vi "AbortMultiple.vi"(8 "error in (no error)":errorcluster, 9 "taskId":i32(ring) items=["TLibrary", "T01", "T02", "T03", "T04", "T05", "T06", "T07", "T08", "T09", "T10", "T11", "T12", "T13", "T14", "T15", "T16", "T17", "T18", "T19", "T20", "T21", "T22", "T23", "T24", "T25", "T26", "T27", "T28", "T29", "T30", "T31"], 10 "axis names":string[](array[string]), 11 "controller in":refnum<k24>) -> (0 "error out":errorcluster, 3 "controller out":refnum<k24>)   [LabVIEW 2016, in "Aerotech VIs.lvlib"]
uses:
  Aerotech VIs.lvlib
  C:/Users/HEP Gantry/Documents/Old Projects/V1 Johan Detector Assembly Project Pre-TypeDef/VIs/Low-Level Instrument VIs/Aerotech/Bin/Aerotech.A3200.LabVIEW.dll
  HEP Gantry/Documents/Old Projects/V1 Johan Detector Assembly Project Pre-TypeDef/VIs/Low-Level Instrument VIs/Aerotech/Bin/Aerotech.A3200.LabVIEW.dll
  C:/Users/HEP Gantry/Documents/Assembly/V4/Drivers/Aerotech A3200/Bin/Aerotech.A3200.dll
  HEP Gantry/Documents/Assembly/V4/Drivers/Aerotech A3200/Bin/Aerotech.A3200.dll
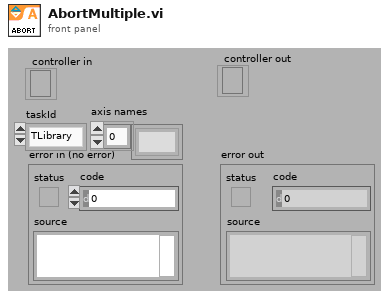
[diagram p1: front panel]
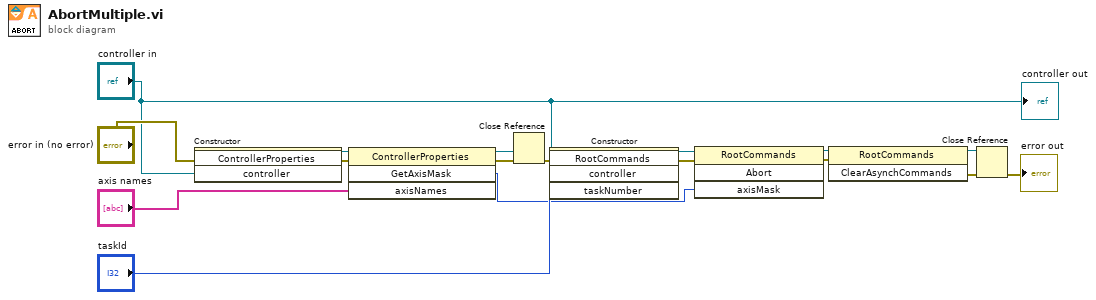
[diagram p0: block diagram]
diagram:
  n1 = constructor class="ControllerProperties"(error in="error in (no error)", "controller"="controller in") -> (reference out=w17:refnum<k24>, error out=w16:errorcluster)  [unwired: 2 in, 2 out]
  n2 = invoke class="ControllerProperties" method="GetAxisMask"(reference=w17, error in=w16, "axisNames"="axis names") -> (reference out=w14:refnum<k24>, error out=w15:errorcluster, "GetAxisMask"=w1:i32)  [unwired: 1 in, 1 out]
  n3 = Close Reference(reference=w14, error in (no error)=w15) -> (error out=w8:errorcluster)
  n4 = constructor class="RootCommands"(error in=w8, "controller"="controller in", "taskNumber"="taskId") -> (reference out=w5:refnum<k24>, error out=w4:errorcluster)  [unwired: 2 in, 3 out]
  n5 = invoke class="RootCommands" method="Abort"(reference=w5, error in=w4, "axisMask"=w1) -> (reference out=w2:refnum<k24>, error out=w6:errorcluster)  [unwired: 1 in, 2 out]
  n6 = invoke class="RootCommands" method="ClearAsynchCommands"(reference=w2, error in=w6) -> (reference out=w10:refnum<k24>, error out=w11:errorcluster)  [unwired: 1 in, 1 out]
  n7 = Close Reference(reference=w10, error in (no error)=w11) -> (error out=→"error out":errorcluster)
  "controller out" <- "controller in"
